vi "Ejemplo5_Bool.vi"() -> ()   [LabVIEW 2020]
panel:
  out "CL A":bool
  out "NOT":bool
  out "XOR":bool
  out "AND":bool
  in  "Boton 1":bool
  in  "Boton 2":bool
  out "OR":bool
  # "Booleanos"
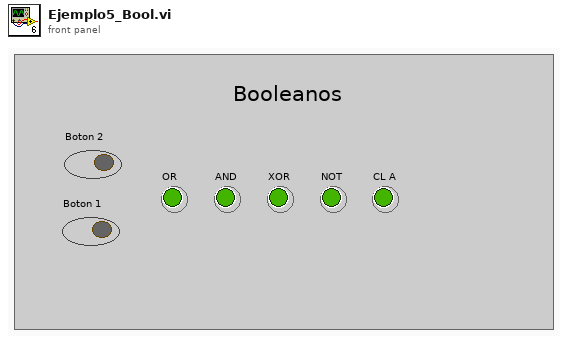
[diagram p1: front panel]
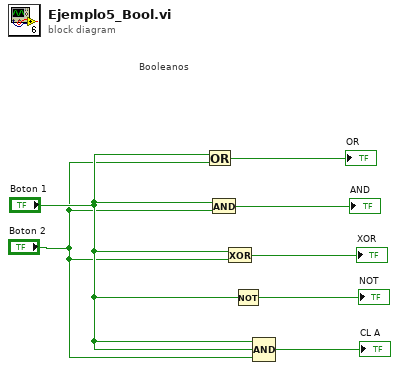
[diagram p0: block diagram]
diagram:
  # "Booleanos"
  n1 = Or(x="Boton 1", y="Boton 2") -> (x .or. y?=→"OR":bool)
  n2 = And(x="Boton 1", y="Boton 2") -> (x .and. y?=→"AND":bool)
  n3 = Exclusive Or(1:"Boton 2", 2:"Boton 1") -> (0:→"XOR":bool)
  n4 = Not(x="Boton 1") -> (.not. x?=→"NOT":bool)
  n5 = Compound Arithmetic op=AND("Boton 1", "Boton 1", "Boton 2") -> (→"CL A":bool)
